vi "OnOff Read.vi"(8 "error in":errorcluster, 11 "Climate Chamber in":refnum<class "Climate Chamber.lvclass">) -> (0 "error out":errorcluster, 1 "Changed or First Call?":bool, 2 "OnOff ACT":bool, 3 "Climate Chamber out":refnum<class "Climate Chamber.lvclass">)   [LabVIEW 2023, in "Climate Chamber.lvclass"]
uses:
  Climate Chamber.lvclass
  Climate Chamber.lvclass/Climate Chamber.ctl
  Low Level Capabilities/OnOff/OnOff.lvclass
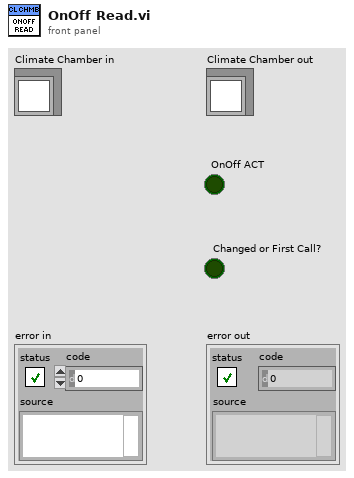
[diagram p1: front panel]
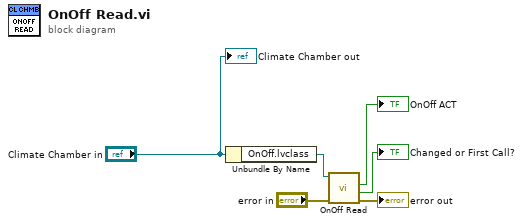
[diagram p0: block diagram]
diagram:
  n1 = Unbundle By Name("Climate Chamber in") -> ("OnOff.lvclass"=w6:refnum<class "OnOff.lvclass">)
  n2 = call-dynamic "OnOff Read.vi"("error in"="error in", "OnOff in"=w6) -> ("error out"=→"error out":errorcluster, "Changed or First Call?"=→"Changed or First Call?":bool, "OnOff ACT"=→"OnOff ACT":bool)  [unwired: 6 in, 1 out]
  "Climate Chamber out" <- "Climate Chamber in"
